vi "QueryNTPparse.vi"(0 "IP Address of NIST Server":string="132.163.4.102", 1 "error in":errorcluster) -> (2 "NTP Time (server time)":u64, 3 "Time stamp string":string, 4 "error out":errorcluster)   [LabVIEW 2012]
panel:
  out "time stamp":timestamp
  out "raw data":string
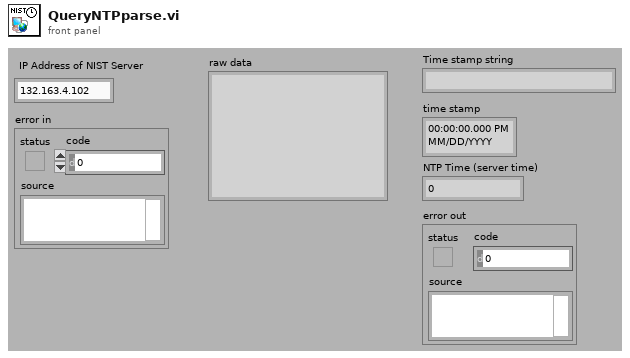
[diagram p1: front panel]
types:
  T1 = cluster{"LI|VM|Mode":u8, "Stratum":u8, "Poll":u8, "Precision":u8, "Root Delay":u32, "Root Dispersion":u32, "Reference Identifier":u32, "Reference Timestamp":fxp<+,64,32>, "Originate Timestamp":fxp<+,64,32>, "Receive Timestamp":fxp<+,64,32>, "Transmit Timestamp":fxp<+,64,32>, "Key Identifier":u32, "Message Digest-1":u64, "Message Digest-2":u64}
  T2 = typedef "LVDateTimeRec.ctl" = cluster{"fractional second":dbl, "second":i32, "minute":i32, "hour":i32, "day of month":i32, "month":i32, "year":i32, "day of week":i32, "day of year":i32, "DST":i32}
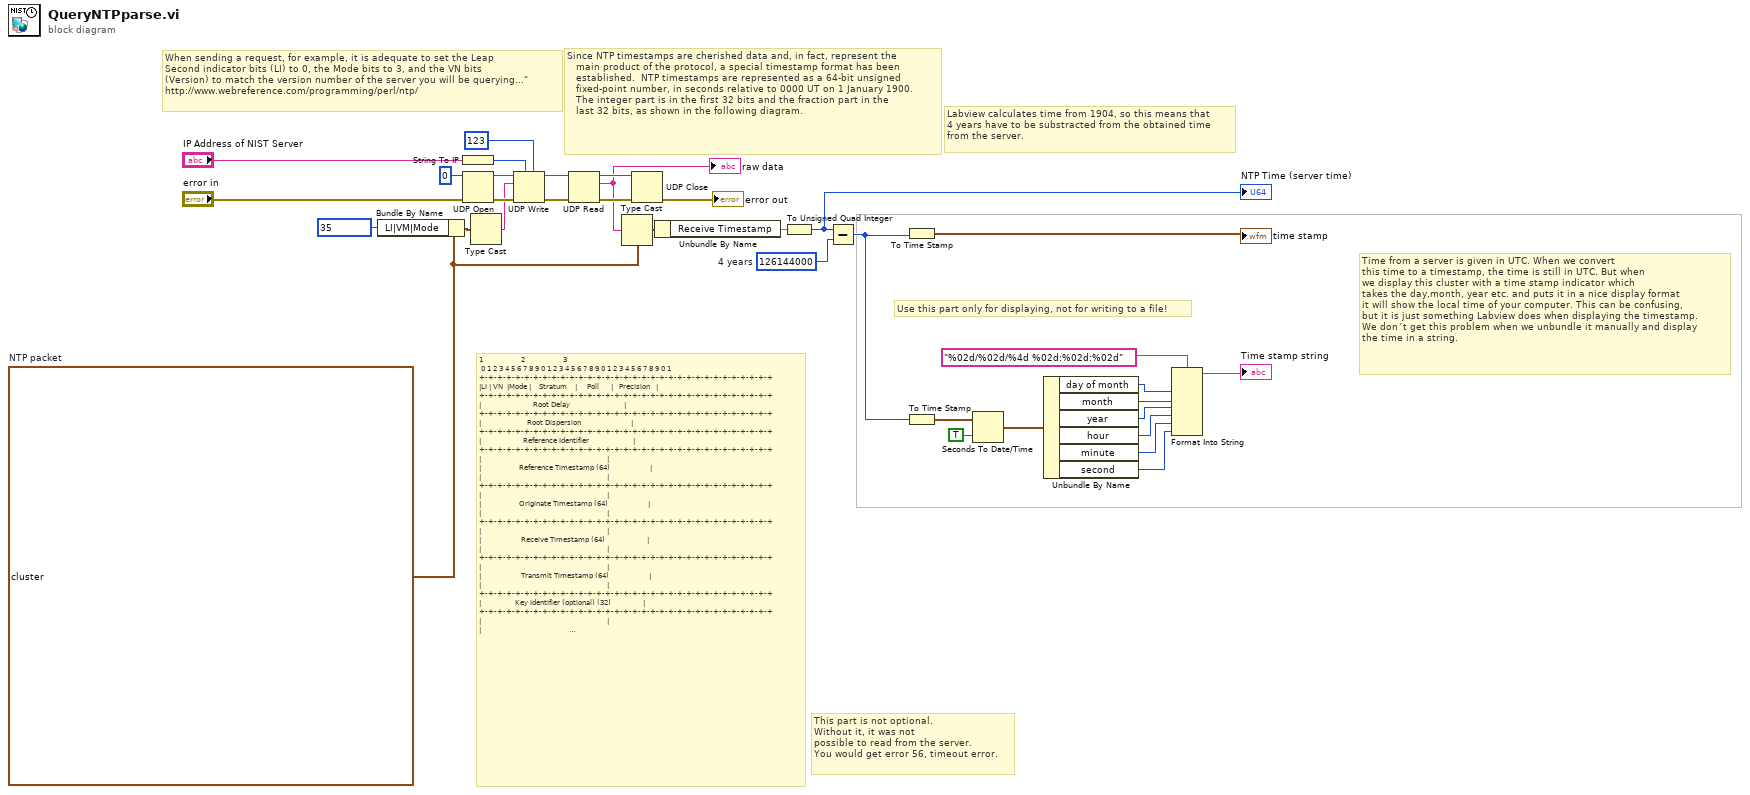
[diagram p0: block diagram]
diagram:
  w15 = T1 {"LI|VM|Mode"=0, "Stratum"=0, "Poll"=0, "Precision"=0, "Root Delay"=0, "Root Dispersion"=0, "Reference Identifier"=0, "Reference Timestamp"=0.0, "Originate Timestamp"=0.0, "Receive Timestamp"=0.0, "Transmit Timestamp"=0.0, "Key Identifier"=0, "Message Digest-1"=0, "Message Digest-2"=0}  # NTP packet
  w16 = u64 126144000  # 4 years
  # "Use this part only for displaying, not for writing to a file!"
  # "Time from a server is given in UTC. When we convert \nthis time to a timestamp, the time is still in UTC. But when\nwe display this cluster with a time stamp indicator which\ntakes the day,month, year etc. and puts it in a nice display format \nit will show the local time of your computer. This can be confusing, \nbut it is just something Labview does when displaying the timestamp.\nWe don´t get this problem when we unbundle it manually and display\nthe time in a string."
  # "This part is not optional.\nWithout it, it was not \npossible to read from the server.\nYou would get error 56, timeout error."
  # "Labview calculates time from 1904, so this means that \n4 years have to be substracted from the obtained time \nfrom the server."
  # "Since NTP timestamps are cherished data and, in fact, represent the\n   main product of the protocol, a special timestamp format has been\n   established.  NTP timestamps are represented as a 64-bit unsigned\n   fixed-point number, in seconds relative to 0000 UT on 1 January 1900.\n   The integer part is in the first 32 bits and the fraction part in the\n   last 32 bits, as shown in the following diagram."
  # "When sending a request, for example, it is adequate to set the Leap\nSecond indicator bits (LI) to 0, the Mode bits to 3, and the VN bits\n(Version) to match the version number of the server you will be querying...\"\nhttp://www.webreference.com/programming/perl/ntp/"
  # "1                   2                   3\n 0 1 2 3 4 5 6 7 8 9 0 1 2 3 4 5 6 7 8 9 0 1 2 3 4 5 6 7 8 9 0 1\n+-+-+-+-+-+-+-+-+-+-+-+-+-+-+-+-+-+-+-+-+-+-+-+-+-+-+-+-+-+-+-+-+\n|LI | VN  |Mode |    Stratum    |     Poll      |   Precision   |\n+-+-+-+-+-+-+-+-+-+-+-+-+-+-+-+-+-+-+-+-+-+-+-+-+-+-+-+-+-+-+-+-+\n|                          Root Delay                           |\n+-+-+-+-+-+-+-+-+-+-+-+-+-+-+-+-+-+-+-+-+-+-+-+-+-+-+-+-+-+-+-+-+\n|                       Root Dispersion                         |\n+-+-+-+-+-+-+-+-+-+-+-+-+-+-+-+-+-+-+-+-+-+-+-+-+-+-+-+-+-+-+-+-+\n|                     Reference Identifier                      |\n+-+-+-+-+-+-+-+-+-+-+-+-+-+-+-+-+-+-+-+-+-+-+-+-+-+-+-+-+-+-+-+-+\n|                                                               |\n|                   Reference Timestamp (64)                    |\n|                                                               |\n+-+-+-+-+-+-+-+-+-+-+-+-+-+-+-+-+-+-+-+-+-+-+-+-+-+-+-+-+-+-+-+-+\n|                                                               |\n|                   Originate Timestamp (64)                    |\n|                                                               |\n+-+-+-+-+-+-+-+-+-+-+-+-+-+-+-+-+-+-+-+-+-+-+-+-+-+-+-+-+-+-+-+-+\n|                                                               |\n|                    Receive Timestamp (64)                     |\n|                                                               |\n+-+-+-+-+-+-+-+-+-+-+-+-+-+-+-+-+-+-+-+-+-+-+-+-+-+-+-+-+-+-+-+-+\n|                                                               |\n|                    Transmit Timestamp (64)                    |\n|                                                               |\n+-+-+-+-+-+-+-+-+-+-+-+-+-+-+-+-+-+-+-+-+-+-+-+-+-+-+-+-+-+-+-+-+\n|                 Key Identifier (optional) (32)                |\n+-+-+-+-+-+-+-+-+-+-+-+-+-+-+-+-+-+-+-+-+-+-+-+-+-+-+-+-+-+-+-+-+\n|                                                               |\n|                                                               |\n|                 Message Digest (optional) (128)               |\n|                                                               |\n|                                                               |\n+-+-+-+-+-+-+-+-+-+-+-+-+-+-+-+-+-+-+-+-+-+-+-+-+-+-+-+-+-+-+-+-+"
  n1 = Bundle By Name(cluster=w15, "LI|VM|Mode"=u8 35) -> (w17:T1)
  n2 = String To IP(1:"IP Address of NIST Server") -> (0:w29:u32)
  n3 = UDP Open(8:"error in", 11:u16 0 ("port")) -> (port=w31:refnum<k16>, 0:w28:errorcluster)  [unwired: 3 in, 1 out]
  n4 = Type Cast(x=w17) -> (*(type *) &x=w24:string)  [unwired: 1 in]
  n5 = UDP Write(address=w29, port or service name=u16 123, connection ID=w31, data in=w24, 8:w28) -> (error out=w27:errorcluster, 3:w32:refnum<k16>)  [unwired: 1 in]
  n6 = UDP Read(connection ID=w32, 8:w27) -> (data out=w21:string, error out=w34:errorcluster, 3:w33:refnum<k16>)  [unwired: 2 in, 2 out]
  "raw data" <- w21
  n7 = Type Cast(type=w15, x=w21) -> (*(type *) &x=w20:T1)
  n8 = UDP Close(connection ID=w33, 8:w34) -> (error out=→"error out":errorcluster)  [unwired: 1 out]
  n9 = Unbundle By Name(w20) -> ("Receive Timestamp"=w19:fxp<+,64,32>)
  n10 = To Unsigned Quad Integer(1:w19) -> (0:w11:u64)
  "NTP Time (server time)" <- w11
  n11 = Subtract(x=w11, y=w16) -> (x-y=w10:u64)
  n12 = To Time Stamp(1:w10) -> (0:→"time stamp":timestamp)
  n13 = To Time Stamp(1:w10) -> (0:w12:timestamp)
  n14 = Seconds To Date/Time(time stamp (now)=w12, to UTC (F)=TRUE) -> (date time rec=w1:T2)
  n15 = Unbundle By Name(w1) -> ("day of month"=w8:i32, "month"=w7:i32, "year"=w6:i32, "hour"=w5:i32, "minute"=w4:i32, "second"=w3:i32)
  n16 = Format Into String(format string="%02d/%02d/%4d %02d:%02d:%02d", w8, w7, w6, w5, w4, w3) -> (resulting string=→"Time stamp string":string)  [unwired: 2 in, 1 out]
